vi "加标体积读取.vi"(7 "是否启用通讯通知":bool, 8 "error in (no error)":errorcluster, 11 "Slave ID":T1) -> (0 "error out":errorcluster, 3 "加标体积":sgl)   [LabVIEW 2016, in "质控单元V1.lvlib"]
uses:
  <vilib>/Plasmionique/MB Master/MB_Master/MB_Master.lvclass
  <vilib>/Plasmionique/MB Master/MB Master.lvlib
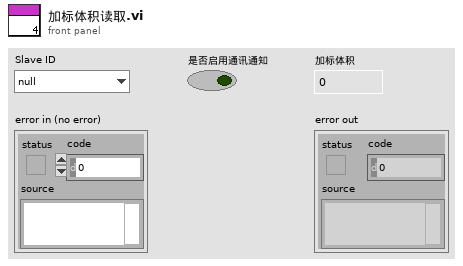
[diagram p1: front panel]
types:
  T1 = typedef "质控单元V1.lvlib/质控slave id.ctl" = enum16{"null", "氨氮", "总磷", "CODMn", "CODCr", "总氮"}
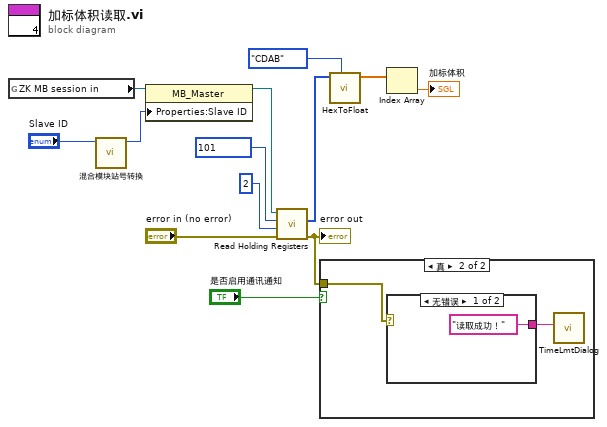
[diagram p0: block diagram]
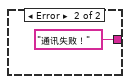
[diagram p3: hidden frame]
diagram:
  n1 = global read "ZK非断电保存全局变量.vi" "ZK MB session in"() -> (w12:refnum<class "MB_Master.lvclass">)
  n2 = call "混合模块站号转换.vi"("Slave ID输入"="Slave ID") -> ("Slave ID输出"=w1:T1)  [unwired: 10 in]
  n3 = property class="MB_Master"(reference=w12, "Properties:Slave ID"=w1) -> (reference out=w10:refnum<class "MB_Master.lvclass">)  [unwired: 1 in, 1 out]
  n4 = call <vilib>:"Read Holding Registers.vi"("error in (no error)"="error in (no error)", "quantity"=u16 2, "starting address"=u16 101, "MB session in"=w10) -> ("error out"=w5:errorcluster, "Registers"=w8:u16[])  [unwired: 5 in, 1 out]
  "error out" <- w5
  n5 = case shown="真" "是否启用通讯通知" {
    tunnel: w5 -> [_ w15]
    frame False {
    }
    frame True {
      n6 = case shown="无错误" w15 {
        tunnel: ["读取成功！" "通讯失败！"] -> w14
        frame No Error {
        }
        frame Error {
        }
      }
      n7 = call "TimeLmtDialog.vi"("Infoin"=w14) -> ()  [unwired: 11 in]
    }
  }
  n8 = call "HexToFloat.vi"("转换类型"=enum16{"DCBA", "CDAB"}."CDAB", "数组"=w8) -> ("FLOAT"=w7:sgl[])  [unwired: 9 in]
  n9 = Index Array(array=w7) -> (element=→"加标体积":sgl)  [unwired: 1 in]
